vi "gentec-M-Link.Queries with String Answers.vi"(0 "VISA resource In":refnum<visa-resource-name>, 2 "Queries with String Answers":T1="VER", 5 "error in (no error)":errorcluster) -> (13 "Read Timeout":bool, 14 "VISA resource Out":refnum<visa-resource-name>, 17 "Answer":string, 19 "error out":errorcluster)   [LabVIEW 2014, in "gentec-M-Link - Driver.lvlib"]
doc: "Data to write: ver, mrd, usn, nam, hvn, ssn, or idn\n\nQueries the firmware version, the maximum reading for the head in use (whatever that is), the user serial number (no idea, what that is), the head version, the head name, the head serial number, or the instrument type."
uses:
  gentec-M-Link - Driver.lvlib
  Type Defs/gentec-M-Link.Queries with String Answers.ctl
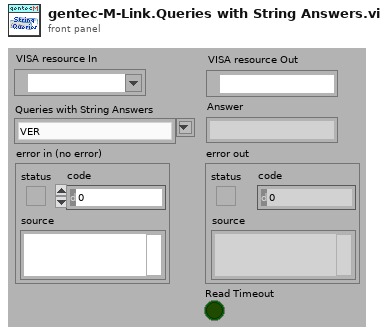
[diagram p1: front panel]
types:
  T1 = typedef "gentec-M-Link - Driver.lvlib/gentec-M-Link.Queries with String Answers.ctl" = string
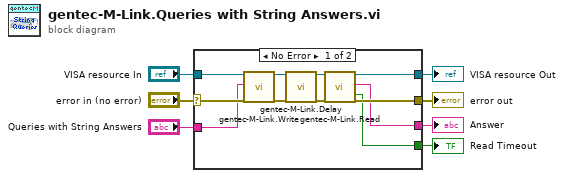
[diagram p0: block diagram]
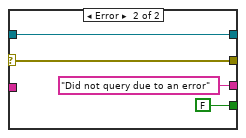
[diagram p2: hidden frame]
diagram:
  n1 = case shown="No Error" "error in (no error)" {
    selector: "error in (no error)" -> [w17 w22]
    tunnel: [w18 w22] -> w6
    tunnel: "VISA resource In" -> [w16 w21]
    tunnel: [w14 w21] -> w4
    tunnel: [w13 "Did not query due to an error" ("Data Read")] -> w3
    tunnel: [w12 FALSE ("Read Timeout")] -> w2
    tunnel: "Queries with String Answers" -> [w8 _]
    frame No Error {
      n2 = call "gentec-M-Link.Write.vi"("VISA resource (In)"=w16, "Data To Write"=w8, "error in (no error)"=w17) -> ("VISA resource (Out)"=w10:refnum<visa-resource-name>, "error out"=w15:errorcluster)  [unwired: 14 in, 1 out]
      n3 = call "gentec-M-Link.Delay.vi"("VISA resource In"=w10, "error in (no error)"=w15) -> ("VISA resource Out"=w9:refnum<visa-resource-name>, "error out"=w11:errorcluster)  [unwired: 16 in]
      n4 = call "gentec-M-Link.Read.vi"("VISA resource (In)"=w9, "error in (no error)"=w11) -> ("VISA resource (Out)"=w14:refnum<visa-resource-name>, "Data Read"=w13:string, "Read Timeout"=w12:bool, "error out"=w18:errorcluster)  [unwired: 13 in, 1 out]
    }
    frame Error {
    }
  }
  "error out" <- w6
  "VISA resource Out" <- w4
  "Answer" <- w3
  "Read Timeout" <- w2
